vi "Write.vi"(6 "Append Index":i32, 8 "error in (no error)":errorcluster, 9 "Notes":string, 10 "Data (Dictionary)":T1[](array[typedef]), 11 "Data.TDMS in":refnum<class "Data.TDMS.lvclass">) -> (0 "error out":errorcluster, 3 "Data.TDMS out":refnum<class "Data.TDMS.lvclass">, 5 "Path out":path)   [LabVIEW 2019, in "Data.TDMS.lvclass"]
uses:
  Data.TDMS.lvclass
  Data/Data.lvclass
  Data/Typedefs/Operation--enum.ctl
  Macros/Conversion.lvclass
  Data/Typedefs/Dictionary--cluster.ctl
  C:/Program Files (x86)/National Instruments/LabVIEW 2020/user.lib/LevyLab/LV to ITX/Data/Data.lvclass
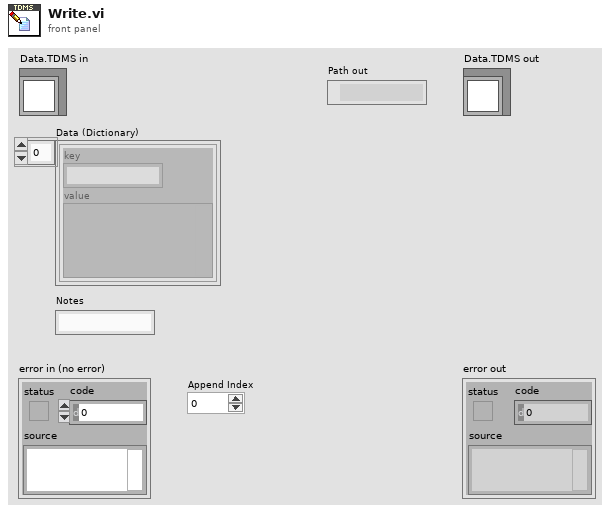
[diagram p1: front panel]
types:
  T1 = typedef "Data.lvclass/Dictionary--cluster.ctl" = cluster{"key":string, "value":variant}
  T2 = typedef "Data.lvclass/Operation--enum.ctl" = enum16{"Read", "Write", "Write + Append"}
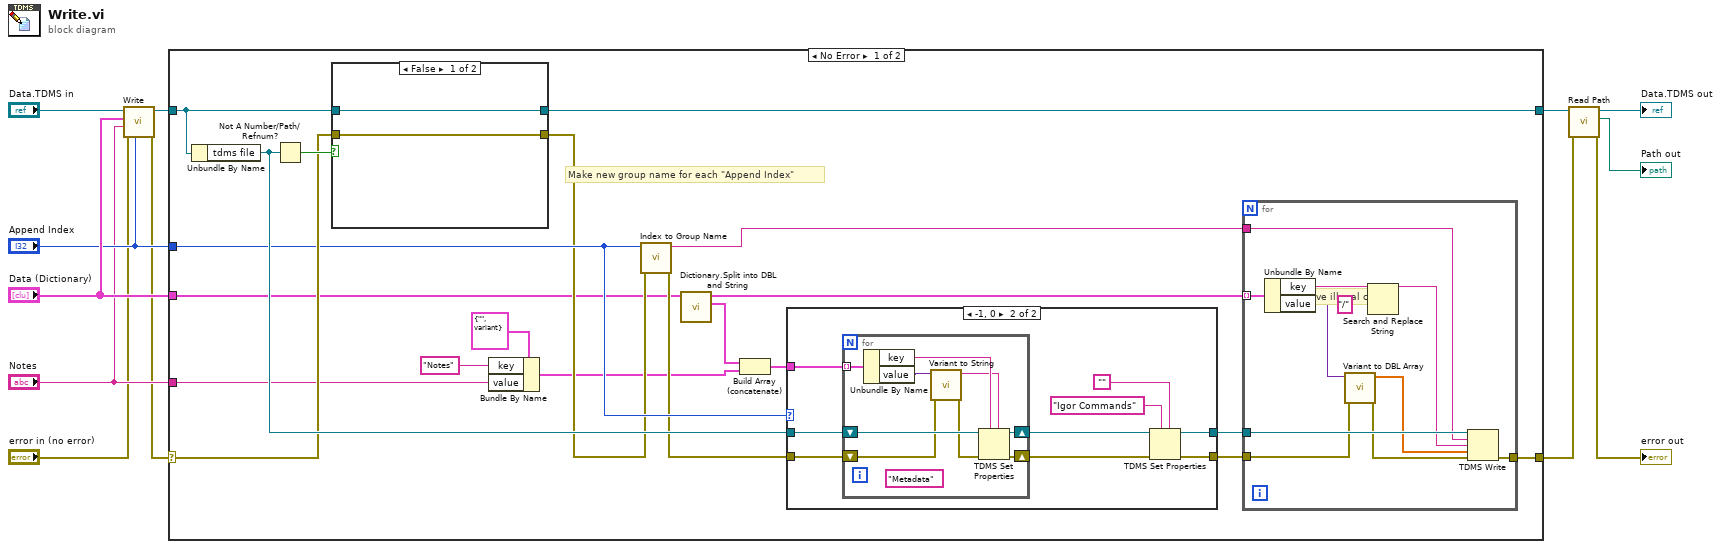
[diagram p0: block diagram]
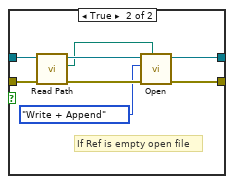
[diagram p2: hidden frame]
diagram:
  n1 = call-parent "Write.vi"("Append Index"="Append Index", "error in (no error)"="error in (no error)", "Notes"="Notes", "Data (Dictionary)"="Data (Dictionary)", "Data in"="Data.TDMS in") -> ("error out"=w1:errorcluster, "Data out"=w6:refnum<class "Data.TDMS.lvclass">)  [unwired: 4 in, 1 out]
  n2 = case shown="No Error" w1 {
    selector: w1 -> [w25 w75]
    tunnel: [w29 w75] -> w10
    tunnel: w6 -> [w32 w74]
    tunnel: [w28 w74] -> w12
    tunnel: "Data (Dictionary)" -> [w20 _]
    tunnel: "Notes" -> [w14 _]
    tunnel: "Append Index" -> [w24 _]
    frame No Error {
      # "Make new group name for each \"Append Index\""
      n3 = Unbundle By Name(w32) -> ("tdms file"=w26:refnum<k34>)
      n4 = Not A Number/Path/Refnum?(number/path/refnum=w26) -> (NaN/Path/Refnum?=w27:bool)
      n5 = case shown="False" w27 {
        tunnel: w32 -> [w33 w42]
        tunnel: [w33 w35] -> w28
        tunnel: [w34 w36] -> w23
        tunnel: w25 -> [w34 w39]
        frame False {
        }
        frame True {
          # "If Ref is empty open file"
          n6 = call "Read Path.vi"("error in (no error)"=w39, "Data Save"=w42) -> ("error out"=w41:errorcluster, "Path"=w38:path, "Data Save out"=w40:refnum<class "Data.TDMS.lvclass">)  [unwired: 7 in]
          n7 = call-dynamic "Open.vi"("Path"=w38, "error in (no error)"=w41, "Operation"=Operation--enum."Write + Append", "Data.TDMS in"=w40) -> ("error out"=w36:errorcluster, "Data.TDMS out"=w35:refnum<class "Data.TDMS.lvclass">)  [unwired: 6 in]
        }
      }
      n8 = Bundle By Name(cluster=T1 {"key"="", "value"=variant} ("input cluster"), "key"="Notes", "value"=w14) -> (w13:T1)
      n9 = call "Index to Group Name.vi"("error in (no error)"=w23, "Append Index"=w24) -> ("error out"=w21:errorcluster, "group name in (Untitled)"=w22:string)  [unwired: 8 in]
      n10 = call "Dictionary.Split into DBL and String.vi"("Data (Dictionary)"=w20) -> ("Data (Dictionary) (String)"=w17:T1[], "Data (Dictionary) (Dbl)"=w19:T1[])  [unwired: 8 in, 1 out]
      n11 = Build Array (concatenate)(w17, w13) -> (w18:T1[])
      n12 = case shown="-1, 0" w24 {
        tunnel: w21 -> [w54 w57]
        tunnel: [w54 w62] -> w31
        tunnel: [w55 w61] -> w30
        tunnel: w26 -> [w55 w58]
        tunnel: w18 -> [_ w56]
        frame Default {
        }
        frame -1, 0 {
          n13 = for {
            shift-right: [w73] -> w64
            shift-left: w58 -> [w71]
            shift-right: [w72] -> w63
            shift-left: w57 -> [w66]
            tunnel: w56 -> [w70] mode=indexing
            (unwired) "Metadata" ("attrib name")
            n14 = Unbundle By Name(w70) -> ("key"=w69:string, "value"=w68:variant)
            n15 = call "Variant to String.vi"("error in (no error)"=w66, "Data (Variant)"=w68) -> ("error out"=w65:errorcluster, "Value"=w67:string)  [unwired: 8 in]
            n16 = TDMS Set Properties(5:w67, 7:w69, 8:w65, 11:w71) -> (0:w72:errorcluster, 3:w73:refnum<k34>)  [unwired: 2 in, 2 out]
          }
          n17 = TDMS Set Properties(5:"", 7:"Igor Commands" ("attrib name"), 8:w63, 11:w64) -> (0:w62:errorcluster, 3:w61:refnum<k34>)  [unwired: 2 in, 2 out]
        }
      }
      n18 = for {
        tunnel: w19 -> [w49] mode=indexing
        tunnel: w31 -> [w47]
        tunnel: w30 -> [w52]
        tunnel: [w51] -> w29
        tunnel: w22 -> [w46]
        # "remove illegal chars"
        n19 = Unbundle By Name(w49) -> ("key"=w50:string, "value"=w45:variant)
        n20 = call "Variant to DBL Array.vi"("error in (no error)"=w47, "Data (Variant)"=w45) -> ("error out"=w48:errorcluster, "1D Array"=w43:dbl[])  [unwired: 7 in, 1 out]
        n21 = Search and Replace String(input string=w50, search string="/") -> (result string=w44:string)  [unwired: 6 in, 3 out]
        n22 = TDMS Write(0:w52, 5:w46, 7:w44, 9:w43, 11:w48) -> (15:w51:errorcluster)  [unwired: 1 in, 3 out]
      }
    }
    frame Error {
    }
  }
  n23 = call "Read Path.vi"("error in (no error)"=w10, "Data Save"=w12) -> ("error out"=→"error out":errorcluster, "Path"=→"Path out":path, "Data Save out"=→"Data.TDMS out":refnum<class "Data.TDMS.lvclass">)  [unwired: 7 in]
